vi "GetType.vi"(8 "error in (no error)":errorcluster, 11 "Configure AM Source [AM] Msg":refnum<class "Configure AM Source [AM] Msg.lvclass">) -> (0 "error out":errorcluster, 2 "Data Sample":variant, 3 "Configure AM Source [AM] Msg":refnum<class "Configure AM Source [AM] Msg.lvclass">)   [LabVIEW 2016, in "CS++Fgen.lvlib" / "Configure AM Source [AM] Msg.lvclass"]
doc: "This VI delivers a sample of the data type format the message expects."
uses:
  Configure AM Source [AM] Msg.lvclass
  Configure AM Source [AM] Msg.lvclass/Configure AM Source [AM] Msg.ctl
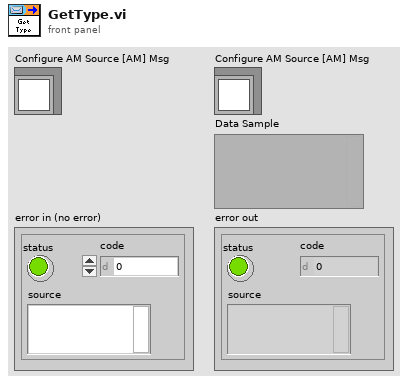
[diagram p1: front panel]
types:
  T1 = cluster{"Channel Name (\"\")":string, "source (Internal)":i32}
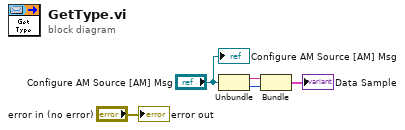
[diagram p0: block diagram]
diagram:
  n1 = Unbundle("Configure AM Source [AM] Msg") -> (w2:string, w1:i32)
  n2 = Bundle("Channel Name (\"\")"=w2, "source (Internal)"=w1) -> (→"Data Sample":T1)  [unwired: 1 in]
  "error out" <- "error in (no error)"
  "Configure AM Source [AM] Msg" <- "Configure AM Source [AM] Msg"
